vi "delete_AI config not UI to UI.vi"(8 "error in (no error)":errorcluster, 11 "AI Config":T2 {"input terminal configuration" items=["default"=-1, "RSE"=10083, "NRSE"=10078, "Differential"=10106, "Pseudodifferential"=12529]; "AI.Coupling" items=["AC"=10045, "DC"=10050, "GND"=10066]}) -> (0 "error out":errorcluster, 1 "DAQ Types":T1[](array[typedef]), 2 "input terminal configurations":i32[](array[numeric]), 3 "AI Config (UI)":T6 {"AI.Coupling" items=["AC"=10045, "DC"=10050, "GND"=10066]})   [LabVIEW 2019, in "Instrument.Lockin.lvclass"]
uses:
  Instrument.Lockin.lvclass
  Instrument.DAQ/Typedefs/AI.config(UI)-array.ctl
  Instrument.DAQ/Typedefs/AI.config(UI)-cluster.ctl
  Instrument.DAQ/Typedefs/AI.coupling-enum.ctl
  Instrument.DAQ/Typedefs/446xAI-enum.ctl
  Instrument.DAQ/Typedefs/AI.config-array.ctl
  Instrument.DAQ/Typedefs/AI.config-cluster.ctl
  Instrument.DAQ/Typedefs/DAQType-enum.ctl
  Instrument.DAQ/Instrument.DAQ.lvclass
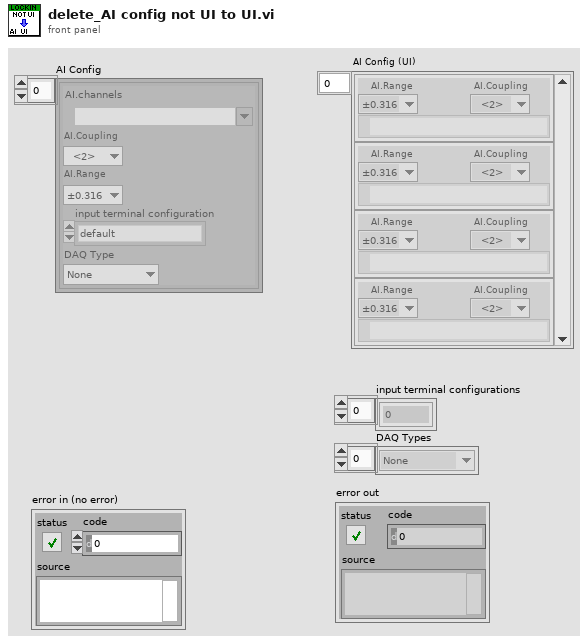
[diagram p1: front panel]
types:
  T1 = typedef "Instrument.DAQ.lvclass/DAQType-enum.ctl" = enum16{"None", "USB 4431", "PXI 446x"}
  T2 = typedef "Instrument.DAQ.lvclass/AI.config-array.ctl" = T3[]
  T3 = typedef "Instrument.DAQ.lvclass/AI.config-cluster.ctl" = cluster{"AI.channels":tag, "AI.Coupling":T4, "AI.Range":T5, "input terminal configuration":i32, "DAQ Type":T1}
  T4 = typedef "Instrument.DAQ.lvclass/AI.coupling-enum.ctl" = u16
  T5 = typedef "Instrument.DAQ.lvclass/446xAI-enum.ctl" = enum16{"±0.316", "±1.00", "±3.16", "±10.0", "±31.6", "±42.4"}
  T6 = typedef "Instrument.DAQ.lvclass/AI.config(UI)-array.ctl" = T7[]
  T7 = typedef "Instrument.DAQ.lvclass/AI.config(UI)-cluster.ctl" = cluster{"AI.Coupling":T4, "AI.channels":tag, "AI.Range":T5}
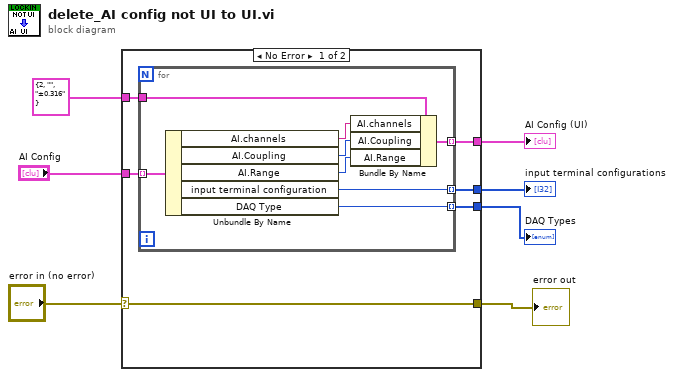
[diagram p0: block diagram]
diagram:
  n1 = case shown="No Error" "error in (no error)" {
    selector: "error in (no error)" -> [w8 w22]
    tunnel: [w13 _] -> w7
    tunnel: "AI Config" -> [w12 _]
    tunnel: T7 {"AI.Coupling"=2, "AI.channels"="", "AI.Range"=enum."±0.316"} ("Cluster") -> [w11 _]
    tunnel: [w10 _] -> w4
    tunnel: [w9 _] -> w3
    tunnel: [w8 w22] -> w1
    frame No Error {
      n2 = for {
        tunnel: w11 -> [w21]
        tunnel: w12 -> [w20] mode=indexing
        tunnel: [w16] -> w13 mode=indexing
        tunnel: [w15] -> w10 mode=indexing
        tunnel: [w14] -> w9 mode=indexing
        n3 = Unbundle By Name(w20) -> ("AI.channels"=w19:tag, "AI.Coupling"=w18:T4, "AI.Range"=w17:T5, "input terminal configuration"=w15:i32, "DAQ Type"=w14:T1)
        n4 = Bundle By Name(cluster=w21, "AI.channels"=w19, "AI.Coupling"=w18, "AI.Range"=w17) -> (w16:T7)
      }
    }
    frame Error {
    }
  }
  "AI Config (UI)" <- w7
  "input terminal configurations" <- w4
  "DAQ Types" <- w3
  "error out" <- w1
